vi "GenerateSine.vi"(0 "GenSpeed Mean":sgl, 5 "GenSpeeed Amplitude":sgl, 7 "2":sgl, 9 "pi":sgl, 11 "frequency (f)":sgl, 12 "time (s)":sgl) -> (4 "Numeric out":sgl)   [LabVIEW 2018]
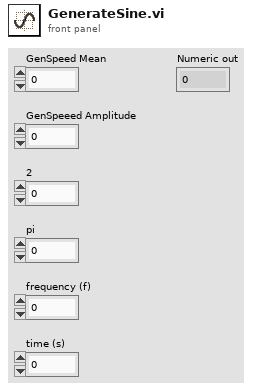
[diagram p1: front panel]
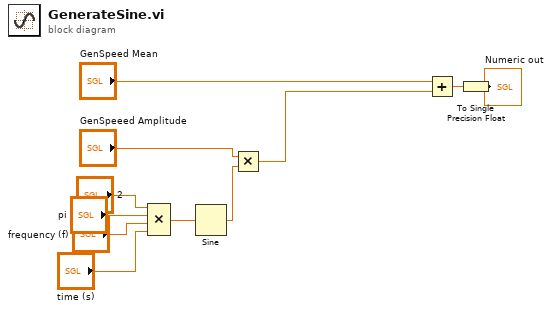
[diagram p0: block diagram]
diagram:
  n1 = Compound Arithmetic op=MULTIPLY("2", "pi", "frequency (f)", "time (s)") -> (w5:sgl)
  n2 = Sine(x=w5) -> (sin(x)=w6:sgl)
  n3 = Multiply(x="GenSpeeed Amplitude", y=w6) -> (x*y=w8:sgl)
  n4 = Add(x="GenSpeed Mean", y=w8) -> (x+y=w10:sgl)
  n5 = To Single Precision Float(number=w10) -> (single precision float=→"Numeric out":sgl)
